vi "Read Data.vi"(8 "error in (no error)":errorcluster, 11 "Test Device in":refnum<class "Test Device.lvclass">) -> (0 "error out":errorcluster, 2 "Base Data Lib:Data":refnum<class "Data.lvclass">, 3 "Test Device out":refnum<class "Test Device.lvclass">)   [LabVIEW 2014, in "Test Device.lvclass"]
uses:
  Test Device.lvclass
  reusable/Data/Data.lvlibp/Data.lvclass
  Test Device.lvclass/Test Device.ctl
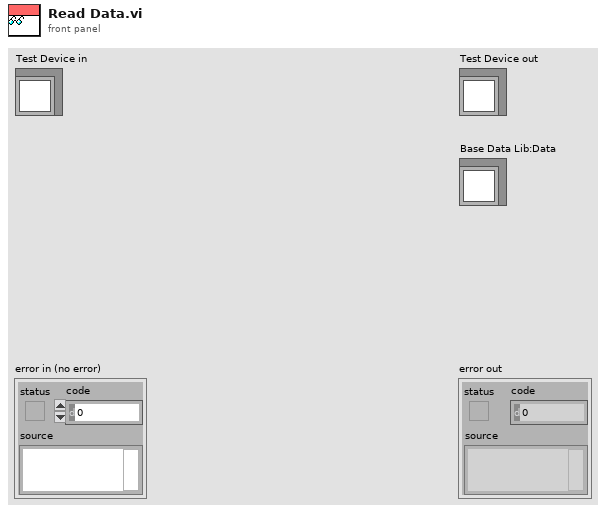
[diagram p1: front panel]
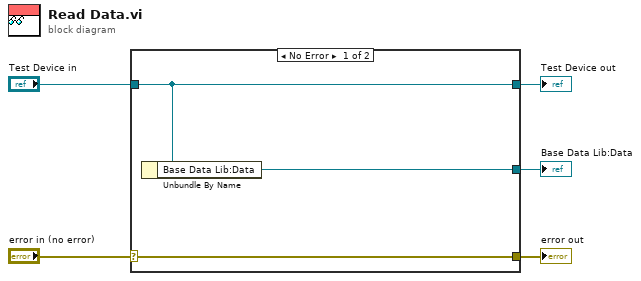
[diagram p0: block diagram]
diagram:
  n1 = case shown="No Error" "error in (no error)" {
    selector: "error in (no error)" -> [w8 w9]
    tunnel: [w8 w9] -> w4
    tunnel: [w7 w10] -> w2
    tunnel: "Test Device in" -> [w7 w10]
    tunnel: [w6 _] -> w1
    frame No Error {
      n2 = Unbundle By Name(w7) -> ("Base Data Lib:Data"=w6:refnum<class "Data.lvclass">)
    }
    frame Error {
    }
  }
  "error out" <- w4
  "Test Device out" <- w2
  "Base Data Lib:Data" <- w1
